vi "Func-엑셀 데이터를 그래프로 출력.vi"() -> ()   [LabVIEW 2015] (continued)
18.962\n22.133\t18.25\t19.031\n22.217\t18.36\t19.1\n22.3\t18.51\t19.166\n22.383\t18.7\t19.23\n22.467\t18.93\t19.297\n22.55\t19.18\t19.367\n22.633\t19.44\t19.432\n22.717\t19.73\t19.496\n22.8\t20\t19.57\n22.883\t20.28\t19.637\n22.967\t20.53\t19.7\n23.05\t20.77\t19.776\n23.133\t20.97\t19.839\n23.217\t21.18\t19.903\n23.3\t21.34\t19.976\n23.383\t21.5\t20.045\n23.467\t21.62\t20.112\n23.55\t21.74\t20.197\n23.633\t21.82\t20.263\n23.717\t21.91\t20.334\n23.8\t21.97\t20.405\n23.883\t22.03\t20.487\n23.967\t22.08\t20.557\n24.05\t22.13\t20.639\n24.133\t22.18\t20.71\n24.217\t22.21\t20.786\n24.3\t22.26\t20.866\n24.383\t22.31\t20.946\n24.467\t22.36\t21.009\n24.55\t22.41\t21.099\n24.633\t22.47\t21.186\n24.717\t22.53\t21.268\n24.8\t22.6\t21.342\n24.883\t22.66\t21.421\n25\t22.73\t21.493\n25\t22.74\t21.5\n25\t22.75\t21.507\n25\t22.75\t21.516\n25\t22.76\t21.521\n25\t22.77\t21.525\n25\t22.78\t21.534\n25\t22.78\t21.545\n25\t22.79\t21.551\n25\t22.8\t21.563\n25\t22.81\t21.57\n25\t22.82\t21.577\n25\t22.83\t21.588\n25\t22.83\t21.594\n25\t22.84\t21.601\n25\t22.85\t21.612\n25\t22.85\t21.62\n25\t22.86\t21.629\n25\t22.88\t21.636\n25\t22.88\t21.644\n25\t22.89\t21.654\n25\t22.9\t21.657\n25\t22.91\t21.666\n25\t22.92\t21.677\n25\t22.92\t21.685\n25\t22.93\t21.693\n25\t22.94\t21.704\n25\t22.95\t21.712\n25\t22.96\t21.719\n25\t22.97\t21.727\n25\t22.98\t21.733\n25\t22.99\t21.741\n25\t23\t21.75\n25\t23.01\t21.757\n25\t23.01\t21.766\n25\t23.02\t21.777\n25\t23.03\t21.788\n25\t23.04\t21.795\n25\t23.05\t21.804\n25\t23.06\t21.813\n25\t23.07\t21.817\n25\t23.07\t21.829\n25\t23.08\t21.836\n25\t23.09\t21.843\n25\t23.1\t21.85\n25\t23.1\t21.857\n25\t23.11\t21.868\n25\t23.11\t21.871\n25\t23.12\t21.875\n25\t23.13\t21.884\n25\t23.14\t21.893\n25\t23.15\t21.904\n25\t23.16\t21.913\n25\t23.17\t21.923\n25\t23.17\t21.931\n25\t23.18\t21.944\n25\t23.19\t21.948\n25\t23.19\t21.952\n25\t23.19\t21.962\n25\t23.2\t21.97\n25\t23.21\t21.978\n25\t23.22\t21.99\n25\t23.23\t21.998\n25\t23.24\t22.005\n25\t23.24\t22.017\n25\t23.25\t22.024\n25\t23.26\t22.034\n25\t23.27\t22.044\n25\t23.28\t22.052\n25\t23.28\t22.06\n25\t23.29\t22.068\n25\t23.29\t22.075\n25\t23.3\t22.082\n25\t23.31\t22.087\n25\t23.31\t22.096\n25\t23.32\t22.104\n25\t23.33\t22.113\n25\t23.34\t22.118\n25\t23.34\t22.124\n25\t23.35\t22.132\n25\t23.36\t22.139\n25\t23.36\t22.149\n25\t23.37\t22.155\n25\t23.37\t22.164\n25\t23.38\t22.173\n25\t23.38\t22.18\n25\t23.4\t22.19\n25\t23.4\t22.203\n25\t23.41\t22.211\n25\t23.42\t22.222\n25\t23.43\t22.236\n25\t23.44\t22.245\n25\t23.44\t22.249\n25\t23.45\t22.255\n25\t23.46\t22.263\n25\t23.46\t22.273\n25\t23.46\t22.279\n25\t23.47\t22.288\n25\t23.48\t22.297\n25\t23.48\t22.303\n25\t23.49\t22.311\n25\t23.49\t22.32\n25\t23.5\t22.327\n25\t23.51\t22.333\n25\t23.52\t22.341\n25\t23.52\t22.352\n25\t23.53\t22.354\n25\t23.54\t22.364\n25\t23.54\t22.373\n25\t23.55\t22.379\n25\t23.55\t22.389\n25\t23.55\t22.396\n25\t23.56\t22.407\n25\t23.56\t22.417\n25\t23.57\t22.427\n25\t23.58\t22.436\n25\t23.59\t22.447\n25\t23.59\t22.452\n25\t23.6\t22.461\n25\t23.61\t22.47\n25\t23.62\t22.476\n25\t23.62\t22.487\n25\t23.63\t22.496\n25\t23.63\t22.508\n25\t23.64\t22.516\n25\t23.64\t22.523\n25\t23.65\t22.528\n25\t23.66\t22.535\n25\t23.66\t22.544\n25\t23.67\t22.549\n25\t23.68\t22.556\n25\t23.69\t22.567\n25\t23.7\t22.577\n25\t23.7\t22.588\n25\t23.71\t22.594\n25\t23.71\t22.604\n25\t23.72\t22.618\n25\t23.73\t22.622\n25\t23.73\t22.629\n25\t23.73\t22.635\n25\t23.74\t22.642\n25\t23.75\t22.645\n25\t23.76\t22.655\n25\t23.76\t22.662\n25\t23.77\t22.67\n25\t23.78\t22.682\n25\t23.79\t22.689\n25\t23.79\t22.701\n25\t23.8\t22.708\n25\t23.81\t22.721\n25\t23.81\t22.735\n25\t23.81\t22.741\n25\t23.82\t22.749\n25\t23.83\t22.759\n25\t23.83\t22.763\n25\t23.84\t22.767\n25\t23.84\t22.776\n25\t23.85\t22.783\n25\t23.86\t22.793\n25\t23.87\t22.803\n25\t23.87\t22.812\n25\t23.88\t22.816\n25\t23.88\t22.822\n25\t23.89\t22.828\n25\t23.89\t22.835\n25\t23.9\t22.847\n25\t23.9\t22.857\n25\t23.9\t22.873\n25\t23.91\t22.882\n25\t23.92\t22.888\n25\t23.92\t22.896\n25\t23.93\t22.902\n25\t23.93\t22.905\n25\t23.94\t22.913\n25\t23.95\t22.92\n25\t23.96\t22.93\n25\t23.97\t22.942\n25\t23.97\t22.954\n25\t23.98\t22.964\n25\t23.99\t22.971\n25\t23.99\t22.98\n25\t23.99\t22.986\n25\t23.99\t22.996\n25\t24\t23\n25\t24.01\t23.006\n25\t24.01\t23.015\n25\t24.02\t23.025\n25\t24.03\t23.034\n25\t24.04\t23.04\n25\t24.05\t23.053\n25\t24.05\t23.066\n25\t24.06\t23.076\n25\t24.07\t23.08\n25\t24.07\t23.092\n25\t24.08\t23.099\n25\t24.08\t23.104\n25\t24.08\t23.113\n25\t24.09\t23.121\n25\t24.09\t23.13\n25\t24.1\t23.14\n25\t24.1\t23.148\n25\t24.11\t23.155\n25\t24.12\t23.163\n25\t24.13\t23.17\n25\t24.13\t23.179\n25\t24.14\t23.188\n25\t24.14\t23.193\n25\t24.15\t23.203\n25\t24.16\t23.214\n25\t24.16\t23.218\n25\t24.17\t23.222\n25\t24.17\t23.233\n25\t24.17\t23.245\n25\t24.17\t23.253\n25\t24.18\t23.263\n25\t24.19\t23.272\n25\t24.2\t23.282\n25\t24.21\t23.291\n25\t24.22\t23.296\n25\t24.22\t23.301\n25\t24.22\t23.312\n25\t24.23\t23.32\n25\t24.23\t23.327\n25\t24.24\t23.335\n25\t24.25\t23.343\n25\t24.26\t23.353\n25\t24.26\t23.359\n25\t24.26\t23.364\n25\t24.27\t23.375\n25\t24.27\t23.381\n25\t24.28\t23.389\n25\t24.28\t23.399\n25\t24.29\t23.405\n25\t24.29\t23.416\n25\t24.3\t23.426\n25\t24.3\t23.436\n25\t24.31\t23.443\n25\t24.31\t23.452\n25\t24.32\t23.46\n25\t24.32\t23.468\n25\t24.33\t23.479\n25\t24.33\t23.486\n25\t24.34\t23.496\n25\t24.34\t23.505\n25\t24.35\t23.513\n25\t24.35\t23.518\n25\t24.35\t23.525\n25\t24.35\t23.532\n25\t24.36\t23.541\n25\t24.37\t23.55\n25\t24.37\t23.562\n25\t24.38\t23.573\n25\t24.38\t23.586\n25\t24.39\t23.594\n25\t24.39\t23.605\n25\t24.39\t23.609\n25\t24.4\t23.618\n25\t24.4\t23.626\n25\t24.41\t23.63\n25\t24.41\t23.638\n25\t24.42\t23.646\n25\t24.42\t23.657\n25\t24.43\t23.662\n25\t24.43\t23.674\n25\t24.44\t23.681\n25\t24.44\t23.685\n25\t24.44\t23.697\n25\t24.44\t23.705\n25\t24.44\t23.714\n25\t24.44\t23.721\n25\t24.45\t23.731\n25\t24.46\t23.739\n25\t24.46\t23.745\n25\t24.47\t23.752\n25\t24.47\t23.756\n25\t24.48\t23.766\n25\t24.48\t23.774\n25\t24.49\t23.786\n25\t24.49\t23.793\n25\t24.5\t23.797\n25\t24.5\t23.807\n25\t24.5\t23.814\n25\t24.51\t23.82\n25\t24.51\t23.832\n25\t24.52\t23.84\n25\t24.52\t23.849\n25\t24.53\t23.859\n25\t24.53\t23.867\n25\t24.53\t23.875\n25\t24.53\t23.884\n25\t24.54\t23.889\n25\t24.54\t23.899\n25\t24.55\t23.912\n25\t24.55\t23.916\n25\t24.55\t23.924\n25\t24.56\t23.934\n25\t24.56\t23.942\n25\t24.57\t23.949\n25\t24.57\t23.959\n25\t24.58\t23.968\n25\t24.58\t23.975\n25\t24.59\t23.984\n25\t24.59\t23.99\n25\t24.59\t23.998\n25\t24.59\t24.006\n25\t24.6\t24.014\n25\t24.6\t24.022\n25\t24.61\t24.035\n25\t24.61\t24.042\n25\t24.62\t24.048\n25\t24.62\t24.059\n25\t24.62\t24.067\n25\t24.62\t24.074\n25\t24.63\t24.082\n25\t24.63\t24.09\n25\t24.63\t24.102\n25\t24.64\t24.106\n25\t24.64\t24.114\n25\t24.64\t24.127\n25\t24.65\t24.134\n25\t24.65\t24.142\n25\t24.65\t24.153\n25\t24.66\t24.165\n25\t24.66\t24.171\n25\t24.66\t24.18\n25\t24.66\t24.186\n25\t24.67\t24.196\n25\t24.67\t24.207\n25\t24.67\t24.213\n25\t24.68\t24.218\n25\t24.68\t24.229\n25\t24.68\t24.236\n25\t24.68\t24.239\n25\t24.69\t24.244\n25\t24.69\t24.249\n25\t24.7\t24.261\n25\t24.7\t24.269\n25\t24.7\t24.275\n25\t24.7\t24.288\n25\t24.71\t24.295\n25\t24.71\t24.301\n25\t24.71\t24.31\n25\t24.71\t24.322\n25\t24.71\t24.331\n25\t24.71\t24.342\n25\t24.72\t24.352\n25\t24.72\t24.362\n25\t24.72\t24.372\n25\t24.72\t24.376\n25\t24.73\t24.386\n25\t24.73\t24.393\n25\t24.73\t24.401\n25\t24.73\t24.407\n25\t24.74\t24.418\n25\t24.74\t24.424\n25\t24.75\t24.425\n25\t24.75\t24.436\n25\t24.76\t24.439\n25\t24.76\t24.448\n25\t24.77\t24.457\n25\t24.77\t24.461\n25\t24.77\t24.475\n25\t24.77\t24.482\n25\t24.77\t24.491\n25\t24.77\t24.501\n25\t24.78\t24.508\n25\t24.78\t24.52\n25\t24.79\t24.53\n25\t24.79\t24.538\n25\t24.79\t24.548\n25\t24.79\t24.554\n25\t24.8\t24.56\n25\t24.8\t24.564\n25\t24.8\t24.575\n25\t24.8\t24.586\n25\t24.8\t24.591\n25\t24.8\t24.6\n25\t24.8\t24.609\n25\t24.81\t24.615\n25\t24.81\t24.626\n25\t24.81\t24.63\n25\t24.81\t24.638\n25\t24.81\t24.65\n25\t24.81\t24.661\n25\t24.82\t24.673\n25\t24.82\t24.681\n25\t24.82\t24.689\n25\t24.83\t24.7\n25\t24.83\t24.708\n25\t24.83\t24.712\n25\t24.83\t24.718\n25\t24.83\t24.723\n25\t24.83\t24.73\n25\t24.84\t24.741\n25\t24.84\t24.746\n25\t24.84\t24.756\n25\t24.85\t24.766\n25\t24.85\t24.777\n25\t24.85\t24.789\n25\t24.85\t24.798\n25\t24.85\t24.803\n25\t24.85\t24.807\n25\t24.85\t24.819\n25\t24.86\t24.825\n25\t24.86\t24.828\n25\t24.86\t24.837\n25\t24.86\t24.848\n25\t24.86\t24.855\n25\t24.87\t24.859\n25\t24.87\t24.863\n25\t24.87\t24.875\n25\t24.87\t24.882\n25\t24.88\t24.888\n25\t24.88\t24.903\n25\t24.88\t24.912\n25\t24.88\t24.922\n25\t24.88\t24.93\n25\t24.88\t24.938\n25\t24.88\t24.947\n25\t24.88\t24.952\n25\t24.89\t24.958\n25\t24.89\t24.967\n25\t24.89\t24.977\n25\t24.89\t24.986\n25\t24.89\t24.991\n25\t24.89\t25\n25\t24.89\t25.009\n25\t24.89\t25.013\n25\t24.89\t25.022\n25\t24.89\t25.025\n25\t24.89\t25.035\n25\t24.89\t25.045\n25\t24.89\t25.052\n25\t24.89\t25.06\n25\t24.9\t25.069\n25\t24.9\t25.079\n25\t24.9\t25.084\n25\t24.9\t25.095\n25\t24.9\t25.101\n25\t24.9\t25.111\n25\t24.9\t25.12\n25\t24.9\t25.125\n25\t24.91\t25.135\n25\t24.91\t25.141\n25\t24.91\t25.147\n25\t24.91\t25.158\n25\t24.91\t25.167\n25\t24.91\t25.177\n25\t24.92\t25.191\n25\t24.92\t25.196\n25\t24.92\t25.203\n25\t24.92\t25.212\n25\t24.93\t25.218\n25\t24.93\t25.223\n25\t24.93\t25.23\n25\t24.93\t25.241\n25\t24.93\t25.251\n25\t24.93\t25.259\n25\t24.93\t25.264\n25\t24.93\t25.271\n25\t24.93\t25.279\n25\t24.93\t25.284\n25\t24.93\t25.288\n25\t24.94\t25.294\n25\t24.95\t25.303\n25\t24.96\t25.313\n25\t24.97\t25.319\n25\t24.98\t25.332\n25\t25\t25.34\n25\t24.98\t25.35\n25\t24.98\t25.358\n25\t24.98\t25.372\n25\t24.98\t25.381\n25\t24.98\t25.38\n25\t24.98\t25.394\n25\t25\t25.402\n25\t24.98\t25.407\n25\t25\t25.415\n25\t25\t25.419\n25\t25\t25.429\n25\t25\t25.436\n25\t25\t25.443\n25\t25\t25.452\n25\t25\t25.462\n25\t25\t25.472\n25\t25\t25.475\n25\t25\t25.486\n25\t25\t25.492\n25\t25\t25.498\n25\t25\t25.505\n25\t25\t25.513\n25\t25\t25.523\n25\t25\t25.533\n25\t25\t25.538\n25\t25\t25.546\n25\t25\t25.554\n25\t25\t25.559\n25\t25\t25.562\n25\t25\t25.569\n25\t25\t25.577\n25\t25\t25.587\n25\t25\t25.597\n25\t25\t25.604\n25\t25\t25.616\n25\t25\t25.625\n25\t25\t25.635\n25\t25\t25.644\n25\t25\t25.654\n25\t25\t25.661\n25\t25\t25.668\n25\t25\t25.676\n25\t25\t25.679\n25\t25\t25.683\n25\t25\t25.69\n25\t25\t25.699\n25\t25\t25.709\n25\t25\t25.716\n25\t25\t25.728\n25\t25\t25.742\n25\t25\t25.747\n25\t25\t25.753\n25\t25\t25.759\n25\t25\t25.765\n25\t25\t25.77\n25\t25\t25.778\n25\t25\t25.784\n25\t25\t25.793\n25\t25\t25.804\n25\t25\t25.811\n25\t25\t25.816\n25\t25\t25.821\n25\t25\t25.834\n25\t25\t25.839\n25\t25\t25.846\n25\t25\t25.857\n25\t25\t25.864\n25\t25\t25.876\n25\t25\t25.878\n25\t25\t25.885\n25\t25\t25.895\n25\t25\t25.901\n25\t25\t25.911\n25\t25\t25.915\n25\t25\t25.923\n25\t25\t25.931\n25\t25\t25.938\n25\t25\t25.944\n25\t25\t25.954\n25\t25\t25.964\n25\t25\t25.97\n25\t25\t25.979\n25\t25\t25.989\n25\t25\t25.996\n25\t25\t26.011\n25\t25\t26.014\n25\t25\t26.022\n25\t25\t26.031\n25\t25\t26.032\n25\t25\t26.043\n25\t25\t26.045\n25\t25\t26.05\n25\t25\t26.057\n25\t25\t26.064\n25\t25\t26.07\n25\t25\t26.072\n25\t25\t26.079\n25\t25\t26.089\n25\t25\t26.093\n25\t25\t26.102\n25\t25\t26.109\n25\t25\t26.118\n25\t25\t26.126\n25\t25\t26.135\n25\t25\t26.145\n25\t25\t26.154\n25\t25\t26.164\n25\t25\t26.168\n25\t25\t26.184\n25\t25\t26.185\n25\t25\t26.192\n25\t25\t26.198\n25\t25\t26.206\n25\t25\t26.218\n25\t25\t26.223\n25\t25\t26.233\n25\t25\t26.241\n25\t25\t26.251\n25\t25\t26.255\n25\t25\t26.263\n25\t25\t26.267\n25\t25\t26.27\n25\t25\t26.278\n25\t25\t26.28\n25\t25\t26.286\n25\t25\t26.295\n25\t25\t26.305\n25\t25\t26.316\n25\t25\t26.324\n25\t25\t26.334\n25\t25\t26.34\n25\t25\t26.352\n25\t25\t26.359\n25\t25\t26.362\n25\t25\t26.375\n25\t25\t26.379\n25\t25\t26.388\n25\t25\t26.392\n25\t25\t26.398\n25\t25\t26.405\n25\t25\t26.414\n25\t25\t26.425\n25\t25\t26.432\n25\t25\t26.44\n25\t25\t26.443\n25\t25\t26.452\n25\t25\t26.457\n25\t25\t26.463\n25\t25\t26.47\n25\t25\t26.48\n25\t25\t26.489\n25\t25\t26.493\n25\t25\t26.504\n25\t25\t26.51\n25\t25\t26.521\n25\t25\t26.524\n25\t25\t26.532\n25\t25\t26.539\n25\t25\t26.546\n25\t25\t26.552\n25\t25\t26.559\n25\t25\t26.568\n25\t25\t26.572\n25\t25\t26.581\n25\t25\t26.586\n25\t25\t26.589\n25\t25\t26.598\n25\t25\t26.602\n25\t25\t26.607\n25\t25\t26.618\n25\t25\t26.626\n25\t25\t26.634\n25\t25\t26.639\n25\t25\t26.647\n25\t25\t26.655\n25\t25\t26.662\n25\t25\t26.664\n25\t25\t26.674\n25\t25\t26.684\n25\t25\t26.687\n25\t25\t26.693\n25\t25\t26.703\n25\t25\t26.712\n25\t25\t26.716\n25\t25\t26.727\n25\t25\t26.737\n25\t25\t26.745\n25\t25\t26.75\n25\t25\t26.757\n25\t25\t26.763\n25\t25\t26.772\n25\t25\t26.777\n25\t25\t26.784\n25\t25\t26.793\n25\t25\t26.799\n25\t25\t26.808\n25\t25\t26.811\n25\t25\t26.816\n25\t25\t26.825\n25\t25\t26.828\n25\t25\t26.832\n25\t25\t26.841\n25\t25\t26.845\n25\t25\t26.852\n25\t25\t26.862\n25\t25\t26.871\n25\t25\t26.88\n25\t25\t26.888\n25\t25\t26.898\n25\t25\t26.904\n25\t25\t26.91\n25\t25\t26.914\n25\t25\t26.921\n25\t25\t26.925\n25\t25\t26.929\n25\t25\t26.936\n25\t25\t26.946\n25\t25\t26.953\n25\t25\t26.961\n25\t25\t26.973\n25\t25\t26.979\n25\t25\t26.982\n25\t25\t26.991\n25\t25\t26.996\n25\t25\t27.004\n25\t25\t27.01\n25\t25\t27.018\n25\t25\t27.03\n25\t25\t27.034\n25\t25\t27.043\n25\t25\t27.05\n25\t25\t27.053\n25\t25\t27.056\n25\t25\t27.07\n25\t25\t27.077\n25\t25\t27.082\n25\t25\t27.09\n25\t25\t27.098\n25\t25\t27.107\n25\t25\t27.108\n25\t25\t27.113\n25\t25\t27.117\n25\t25\t27.124\n25\t25\t27.13\n25\t25\t27.135\n25\t25\t27.145\n25\t25\t27.152\n25\t25\t27.162\n25\t25\t27.169\n25\t25\t27.174\n25\t25\t27.181\n25\t25\t27.189\n25\t25\t27.196\n25\t25\t27.206\n25\t25\t27.216\n25\t25\t27.221\n25\t25\t27.229\n25\t25\t27.232\n25\t25\t27.239\n25\t25\t27.245\n25\t25\t27.246\n25\t25\t27.252\n25\t25\t27.261\n25\t25\t27.267\n25\t25\t27.27\n25\t25\t27.279\n25\t25\t27.287\n25\t25\t27.297\n25\t25\t27.304\n25\t25\t27.309\n25\t25\t27.314\n25\t25\t27.322\n25\t25\t27.327\n25\t25\t27.33\n25\t25\t27.341\n25\t25\t27.349\n25\t25\t27.355\n25\t25\t27.363\n25\t25\t27.369\n25\t25\t27.375\n25\t25\t27.379\n25\t25\t27.385\n25\t25\t27.393\n25\t25\t27.398\n25\t25\t27.404\n25\t25\t27.41\n25\t25\t27.417\n25\t25\t27.421\n25\t25\t27.425\n25\t25\t27.431\n25\t25\t27.435\n25\t25\t27.443\n25\t25\t27.446\n25\t25\t27.458\n25\t25\t27.469\n25\t25\t27.475\n25\t25\t27.482\n25\t25\t27.49\n25\t25\t27.498\n25\t25\t27.5\n25\t25\t27.508\n25\t25\t27.514\n25\t25\t27.521\n25\t25\t27.532\n25\t25\t27.54\n25\t25\t27.545\n25\t25\t27.55\n25\t25\t27.557\n25\t25\t27.563\n25\t25\t27.57\n25\t25\t27.571\n25\t25\t27.576\n25\t25\t27.587\n25\t25\t27.593\n25\t25\t27.597\n25\t25\t27.602\n25\t25\t27.609\n25\t25\t27.618\n25\t25\t27.622\n25\t25\t27.626\n25\t25\t27.634\n25\t25\t27.638\n25\t25\t27.646\n25\t25\t27.654\n25\t25\t27.658\n25\t25\t27.666\n25\t25\t27.676\n25\t25\t27.684\n25\t25\t27.688\n25\t25\t27.696\n25\t25\t27.704\n25\t25\t27.705\n25\t25\t27.713\n25\t25\t27.718\n25\t25\t27.723\n25\t25\t27.729\n25\t25\t27.735\n25\t25\t27.743\n25\t25\t27.75\n25\t25\t27.755\n25\t25\t27.763\n25\t25\t27.77\n25\t25\t27.774\n25\t25\t27.779\n25\t25\t27.782\n25\t25\t27.786\n25\t25\t27.788\n25\t25\t27.794\n25\t25\t27.799\n25\t25\t27.805\n25\t25\t27.813\n25\t25\t27.818\n25\t25\t27.825\n25\t25\t27.836\n25\t25\t27.842\n25\t25\t27.846\n25\t25\t27.858\n25\t25\t27.868\n25\t25\t27.872\n25\t25\t27.878\n25\t25\t27.882\n25\t25\t27.887\n25\t25\t27.893\n25\t25\t27.895\n25\t25\t27.904\n25\t25\t27.909\n25\t25\t27.914\n25\t25\t27.923\n25\t25\t27.925\n25\t25\t27.935\n25\t25\t27.943\n25\t25\t27.945\n25\t25\t27.954\n25\t25\t27.958\n25\t25\t27.966\n25\t25\t27.971\n25\t25\t27.974\n25\t25\t27.984\n25\t25\t27.99\n25\t25\t28\n25\t25\t28.004\n25\t25\t28.007\n25\t25\t28.017\n25\t25\t28.024\n25\t25\t28.027\n25\t25\t28.036\n25\t25\t28.041\n25\t25\t28.048\n25\t25\t28.055\n25\t25\t28.057\n25\t25\t28.063\n25\t25\t28.069\n25\t25\t28.073\n25\t25\t28.075\n25\t25\t28.082\n25\t25\t28.091\n25\t25\t28.096\n25\t25\t28.102\n25\t25\t28.108\n25\t25\t28.115\n25\t25\t28.121\n25\t25\t28.121\n25\t25\t28.127\n25\t25\t28.129\n25\t25\t28.138\n25\t25\t28.149\n25\t25\t28.156\n25\t25\t28.162\n25\t25\t28.172\n25\t25\t28.179\n25\t25\t28.179\n25\t25\t28.181\n25\t25\t28.185\n25\t25\t28.193\n25\t25\t28.198\n25\t25\t28.202\n25\t25\t28.207\n25\t25\t28.213\n25\t25\t28.217\n25\t25\t28.221\n25\t25\t28.232\n25\t25\t28.242\n25\t25\t28.248\n25\t25\t28.261\n25\t25\t28.265\n25\t25\t28.269\n25\t25\t28.272\n25\t25\t28.276\n25\t25\t28.281\n25\t25\t28.286\n25\t25\t28.293\n25\t25\t28.3\n25\t25\t28.308\n25\t25\t28.311\n25\t25\t28.32\n25\t25\t28.323\n25\t25\t28.327\n25\t25\t28.331\n25\t25\t28.333\n25\t25\t28.339\n25\t25\t28.345\n25\t25\t28.349\n25\t25\t28.356\n25\t25\t28.365\n25\t25\t28.373\n25\t25\t28.374\n25\t25\t28.382\n25\t25\t28.388\n25\t25\t28.391\n25\t25\t28.395\n25\t25\t28.398\n25\t25\t28.406\n25\t25\t28.413\n25\t25\t28.415\n25\t25\t28.42\n25\t25\t28.428\n25\t25\t28.435\n25\t25\t28.438\n25\t25\t28.445\n25\t25\t28.454\n25\t25\t28.458\n25\t25\t28.469\n25\t25\t28.469\n25\t25\t28.475\n25\t25\t28.478\n25\t25\t28.481\n25\t25\t28.487\n25\t25\t28.492\n25\t25\t28.502\n25\t25\t28.51\n25\t25\t28.516\n25\t25\t28.521\n25\t25\t28.527\n25\t25\t28.531\n25\t25\t28.534\n25\t25\t28.539\n25\t25\t28.545\n25\t25\t28.548\n25\t25\t28.553\n25\t25\t28.557\n25\t25\t28.561\n25\t25\t28.572\n25\t25\t28.573\n25\t25\t28.58\n25\t25\t28.591\n25\t25\t28.597\n25\t25\t28.602\n25\t25\t28.604\n25\t25\t28.611\n25\t25\t28.614\n25\t25\t28.618\n25\t25\t28.621\n25\t25\t28.625\n25\t25\t28.633\n25\t25\t28.638\n25\t25\t28.645\n25\t25\t28.648\n25\t25\t28.654\n25\t25\t28.661\n25\t25\t28.663\n25\t25\t28.668\n25\t25\t28.671\n25\t25\t28.678\n25\t25\t28.682\n25\t25\t28.686\n25\t25\t28.694\n25\t25\t28.699\n25\t25\t28.707\n25\t25\t28.713\n25\t25\t28.718\n25\t25\t28.726\n25\t25\t28.73\n25\t25\t28.734\n25\t25\t28.741\n25\t25\t28.747\n25\t25\t28.752\n25\t25\t28.755\n25\t25\t28.761\n25\t25\t28.767\n25\t25\t28.777\n25\t25\t28.784\n25\t25\t28.79\n25\t25\t28.798\n25\t25\t28.801\n25\t25\t28.805\n25\t25\t28.809\n25\t25\t28.806\n25\t25\t28.811\n25\t25\t28.818\n25\t25\t28.822\n25\t25\t28.826\n25\t25\t28.83\n25\t25\t28.837\n25\t25\t28.843\n25\t25\t28.847\n25\t25\t28.851\n25\t25\t28.855\n25\t25\t28.858\n25\t25\t28.864\n25\t25\t28.873\n25\t25\t28.877\n25\t25\t28.882\n25\t25\t28.888\n25\t25\t28.893\n25\t25\t28.894\n25\t25\t28.897\n25\t25\t28.9\n25\t25\t28.906\n25\t25\t28.916\n25\t25\t28.922\n25\t25\t28.927\n25\t25\t28.931\n25\t25\t28.936\n25\t25\t28.939\n25\t25\t28.946\n25\t25\t28.951\n25\t25\t28.956\n25\t25\t28.964\n25\t25\t28.969\n25\t25\t28.975\n25\t25\t28.977\n25\t25\t28.979\n25\t25\t28.984\n25\t25\t28.991\n25\t25\t28.998\n25\t25\t29.004\n25\t25\t29.009\n25\t25\t29.013\n25\t25\t29.016\n25\t25\t29.021\n25\t25\t29.025\n25\t25\t29.029\n25\t25\t29.039\n25\t25\t29.043\n25\t25\t29.05\n25\t25\t29.057\n25\t25\t29.061\n25\t25\t29.064\n25\t25\t29.067\n25\t25\t29.074\n25\t25\t29.079\n25\t25\t29.082\n25\t25\t29.084\n25\t25\t29.089\n25\t25\t29.095\n25\t25\t29.096\n25\t25\t29.102\n25\t25\t29.104\n25\t25\t29.107\n25\t25\t29.112\n25\t25\t29.117\n25\t25\t29.125\n25\t25\t29.132\n25\t25\t29.136\n25\t25\t29.142\n25\t25\t29.15\n25\t25\t29.152\n25\t25\t29.155\n25\t25\t29.159\n25\t25\t29.166\n25\t25\t29.17\n25\t25\t29.177\n25\t25\t29.182\n25\t25\t29.188\n25\t25\t29.193\n25\t25\t29.199\n25\t25\t29.204\n25\t25\t29.21\n25\t25\t29.211\n25\t25\t29.215\n25\t25\t29.22\n25\t25\t29.223\n25\t25\t29.229\n25\t25\t29.23\n25\t25\t29.238\n25\t25\t29.246\n25\t25\t29.248\n25\t25\t29.251\n25\t25\t29.256\n25\t25\t29.261\n25\t25\t29.263\n25\t25\t29.267\n25\t25\t29.268\n25\t25\t29.275\n25\t25\t29.282\n25\t25\t29.288\n25\t25\t29.295\n25\t25\t29.304\n25\t25\t29.311\n25\t25\t29.312\n25\t25\t29.316\n25\t25\t29.319\n25\t25\t29.321\n25\t25\t29.325\n25\t25\t29.33\n25\t25\t29.338\n25\t25\t29.341\n25\t25\t29.347\n25\t25\t29.349\n25\t25\t29.354\n25\t25\t29.357\n25\t25\t29.361\n25\t25\t29.368\n25\t25\t29.367\n25\t25\t29.372\n25\t25\t29.375\n25\t25\t29.38\n25\t25\t29.386\n25\t25\t29.393\n25\t25\t29.397\n25\t25\t29.404\n25\t25\t29.407\n25\t25\t29.411\n25\t25\t29.415\n25\t25\t
